vi "保存mes.vi"(11 "参数值":T1(array[cluster])) -> ()   [LabVIEW 2015]
uses:
  Global.vi
  <vilib>/Utility/file.llb/Write Delimited Spreadsheet (string).vi
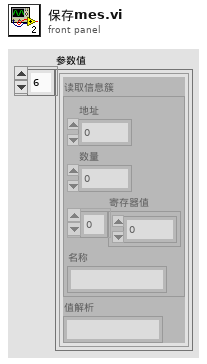
[diagram p1: front panel]
types:
  T1 = cluster{"读取信息簇":cluster{"地址":u16, "数量":u16, "寄存器值":u16[], "名称":string}, "值解析":string}[]
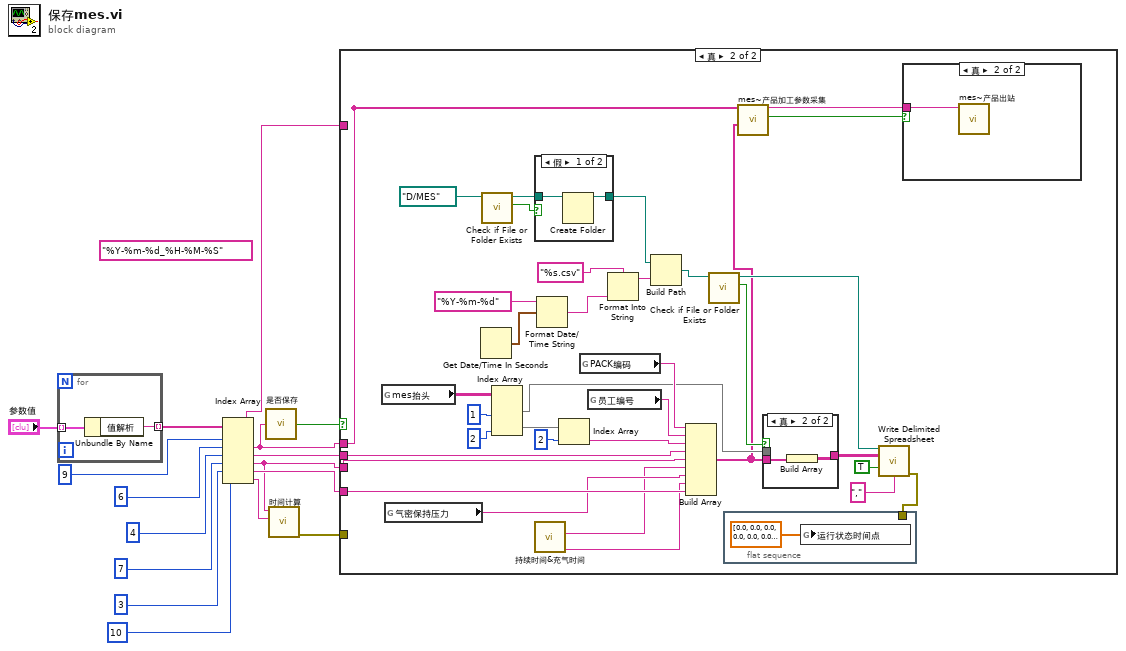
[diagram p0: block diagram]
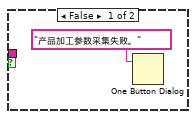
[diagram p3: hidden frame]
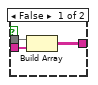
[diagram p4: hidden frame]
diagram:
  (unwired) "%Y-%m-%d_%H-%M-%S" ("时间格式字符串(%c)")
  n1 = for {
    tunnel: "参数值" -> [w18] mode=indexing
    tunnel: [w17] -> w15 mode=indexing
    n2 = Unbundle By Name(w18) -> ("值解析"=w17:string)
  }
  n3 = Index Array(array=w15, index #1=9 ("索引"), index #2=6 ("索引"), index #3=4 ("索引"), index #4=7 ("索引"), index #5=3 ("索引"), index #6=10 ("索引")) -> (element #1=w1:string, element #2=w10:string, element #3=w9:string, element #4=w5:string, element #5=w8:string, element #6=w4:string)
  n4 = call "是否保存.vi"("测试结果"=w10) -> ("保存"=w7:bool)
  n5 = call "时间计算.vi"("运行状态"=w4, "实时压力"=w5) -> ("错误常量out"=w3:errorcluster)  [unwired: 9 in]
  n6 = case shown="真" w7 {
    tunnel: w10 -> [_ w21]
    tunnel: w9 -> [_ w39]
    tunnel: w5 -> [_ w38]
    tunnel: w8 -> [_ w37]
    tunnel: w3 -> [_ _]
    tunnel: w1 -> [_ _]
    frame False {
    }
    frame True {
      n7 = global read "Global.vi" "mes抬头"() -> (w47:string[][])
      n8 = global read "Global.vi" "气密保持压力"() -> (w25:string)
      n9 = Get Date/Time In Seconds() -> (seconds since 1Jan1904=w51:timestamp)
      n10 = call <vilib>:"Check if File or Folder Exists.vi"("path"=path "D:/MES" ("路径")) -> ("file or folder exists?"=w33:bool, "dup path"=w32:path)  [unwired: 8 in, 1 out]
      n11 = Index Array(array=w47, index (col) #1=1 ("禁用的索引 (列)"), index (col) #2=2 ("禁用的索引 (列)")) -> (element #1=w36:string[], element #2=w44:string[])  [unwired: 2 in]
      n12 = case shown="假" w33 {
        tunnel: w32 -> [w62 w63]
        tunnel: [w61 w63] -> w29
        frame False {
          n13 = Create Folder(path (use dialog)=w62) -> (created path=w61:path)  [unwired: 2 in, 2 out]
        }
        frame True {
        }
      }
      n14 = call "持续时间&充气时间.vi"() -> ("气密保持压力持续时间"=w22:string, "气密充气时间"=w23:string)  [unwired: 10 in]
      n15 = Format Date/Time String(time format string (%c)="%Y-%m-%d" ("时间格式字符串(%c)"), seconds (now)=w51) -> (date/time string=w49:string)  [unwired: 1 in]
      n16 = Index Array(array=w44, index=2 ("索引")) -> (element=w40:string)
      n17 = global read "Global.vi" "PACK编码"() -> (w42:string)
      n18 = global read "Global.vi" "员工编号"() -> (w41:string)
      n19 = Format Into String(format string="%s.csv" ("格式字符串"), w49) -> (resulting string=w48:string)  [unwired: 2 in, 1 out]
      n20 = Build Path(base path=w29, name or relative path=w48) -> (appended path=w28:path)
      n21 = Build Array(w42, w41, w40, w39, w38, w23, w25, w22, w37) -> (w20:string[])
      n22 = call <vilib>:"Check if File or Folder Exists.vi"("path"=w28) -> ("file or folder exists?"=w27:bool, "dup path"=w26:path)  [unwired: 8 in, 1 out]
      n23 = flat-sequence {
        tunnel: w24 -> [_]
        frame #0 {
          n24 = global write "Global.vi" "运行状态时间点"(dbl[] [0.0, 0.0, 0.0, 0.0, 0.0, 0.0, 0.0, 0.0, 0.0] ("运行状态时间点")) -> ()
        }
      }
      n25 = call "mes~产品加工参数采集.vi"("采集项"=w20, "测试结果"=w21) -> ("加工参数采集成功"=w19:bool)  [unwired: 8 in, 1 out]
      n26 = case shown="真" w27 {
        tunnel: w36 -> [w58 _]
        tunnel: w20 -> [w57 w60]
        tunnel: [w56 w59] -> w35
        frame False {
          n27 = Build Array(w58, w57) -> (w56:string[][])
        }
        frame True {
          n28 = Build Array(w60) -> (w59:string[][])
        }
      }
      n29 = call-poly <vilib>:"Write Delimited Spreadsheet.vi"("file path (dialog if empty)"=w26, "2D data"=w35, "append to file? (F)"=TRUE, "delimiter (\\t)"="," ("delimiter (\\t)")) -> ("error out"=w24:errorcluster)  [unwired: 10 in, 1 out]
      n30 = case shown="真" w19 {
        tunnel: w21 -> [_ w54]
        frame False {
          n31 = One Button Dialog(message="产品加工参数采集失败。") -> ()  [unwired: 1 in, 1 out]
        }
        frame True {
          n32 = call "mes~产品出站.vi"("测试结果"=w54) -> ()  [unwired: 9 in, 2 out]
        }
      }
    }
  }
